vi "Charger_Enable.vi"(6 "error in":errorcluster, 9 "Charger":T1={"address"="COM8", "position"=3, "setpoint"=7500.0} {"setpoint" min=0.0 max=20000.0 step=100.0; "position" min=0 max=5 step=1}) -> (0 "error out":errorcluster)   [LabVIEW 2020]
uses:
  Charger_Input Control.ctl
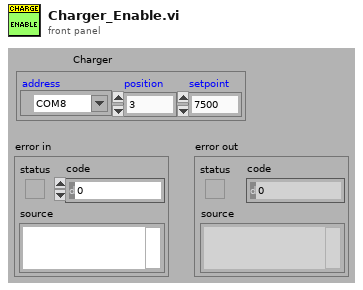
[diagram p1: front panel]
types:
  T1 = typedef "Charger_Input Control.ctl" = cluster{"address":refnum<visa-resource-name>, "position":i32, "setpoint":dbl}
  T2 = enum16{"Disable", "Enable", "Update", "Get Info"}
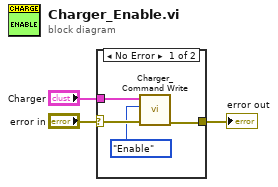
[diagram p0: block diagram]
diagram:
  n1 = case shown="No Error" "error in" {
    selector: "error in" -> [w7 w8]
    tunnel: [w6 w8] -> w3
    tunnel: "Charger" -> [w4 _]
    frame No Error {
      n2 = call "Charger_Command Write.vi"("error in"=w7, "Command"=T2."Enable", "Charger"=w4) -> ("error out"=w6:errorcluster)  [unwired: 5 in, 1 out]
    }
    frame Error {
    }
  }
  "error out" <- w3
